vi "I2C Read Byte.vi"(8 "error in (no error)":errorcluster, 10 "Command":u8 format="%.0x", 11 "LINX I2C in":refnum<class "LINX I2C.lvclass">) -> (0 "error out":errorcluster, 2 "Byte Read":u8, 3 "LINX I2C out":refnum<class "LINX I2C.lvclass">)   [LabVIEW 2020, in "LINX I2C.lvclass"]
uses:
  LINX I2C.lvclass
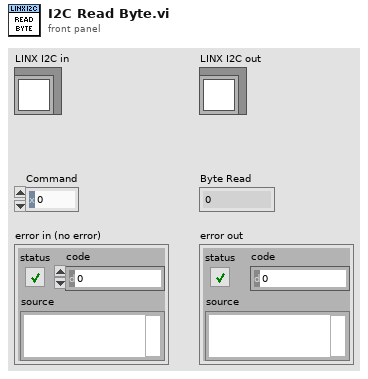
[diagram p1: front panel]
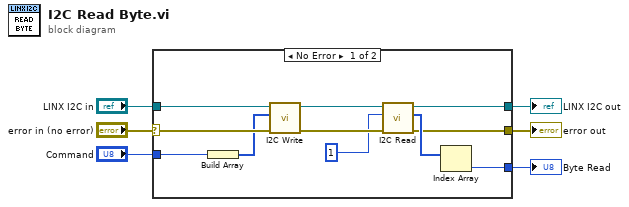
[diagram p0: block diagram]
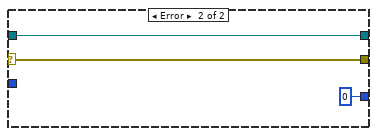
[diagram p2: hidden frame]
diagram:
  n1 = case shown="No Error" "error in (no error)" {
    selector: "error in (no error)" -> [w10 w19]
    tunnel: "Command" -> [w17 _]
    tunnel: [w16 u8 0 ("I2C Slave Address 2")] -> w5
    tunnel: [w14 w19] -> w4
    tunnel: [w12 w20] -> w3
    tunnel: "LINX I2C in" -> [w9 w20]
    frame No Error {
      n2 = Build Array(w17) -> (w8:u8[])
      n3 = call "I2C Write.vi"("error in (no error)"=w10, "Bytes to Write"=w8, "LINX I2C in"=w9) -> ("error out"=w13:errorcluster, "LINX I2C out"=w11:refnum<class "LINX I2C.lvclass">)  [unwired: 7 in]
      n4 = call-dynamic "I2C Read.vi"("error in (no error)"=w13, "# Bytes to Read"=u8 1, "LINX I2C in"=w11) -> ("error out"=w14:errorcluster, "Bytes Read"=w15:u8[], "LINX I2C out"=w12:refnum<class "LINX I2C.lvclass">)  [unwired: 6 in]
      n5 = Index Array(array=w15) -> (element=w16:u8)  [unwired: 1 in]
    }
    frame Error {
    }
  }
  "Byte Read" <- w5
  "error out" <- w4
  "LINX I2C out" <- w3
